vi "Destroy.vi"(8 "Error In":errorcluster, 11 "reference in":refnum<class "BreakfastMenuIterator.lvclass">) -> (0 "Error Out":errorcluster, 3 "reference out":refnum<class "BreakfastMenuIterator.lvclass">)   [LabVIEW 2020, in "BreakfastMenuIterator.lvclass"]
uses:
  BreakfastMenuIterator.lvclass
  BreakfastMenuIterator.lvclass/BreakfastMenuIterator.ctl
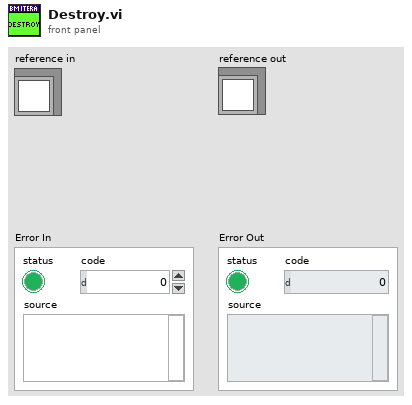
[diagram p1: front panel]
types:
  T1 = typedef "BreakfastMenuIterator.lvclass/ObjectAttributes.ctl" = cluster{"_count":i32, "_items":variant[]}
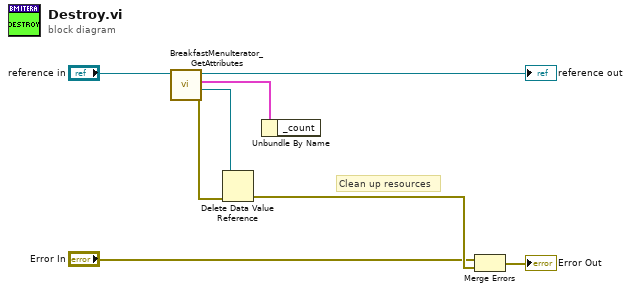
[diagram p0: block diagram]
diagram:
  # "Clean up resources"
  n1 = call "BreakfastMenuIterator_GetAttributes.vi"("reference in"="reference in") -> ("error out"=w5:errorcluster, "DataRef"=w4:refnum<data-value>, "Data"=w3:T1, "reference out"=→"reference out":refnum<class "BreakfastMenuIterator.lvclass">)  [unwired: 7 in]
  n2 = Delete Data Value Reference(data value reference=w4, error in=w5) -> (error out=w2:errorcluster)  [unwired: 1 out]
  n3 = Unbundle By Name(w3) -> ()  [unwired: 1 out]
  n4 = Merge Errors("Error In", w2) -> (→"Error Out":errorcluster)
